vi "PCert-Container-LaunchGlobalDBActor.vi"(8 "error in (no error)":errorcluster, 11 "ERP-Container-UI in":refnum<class "PCert-Container-UI.lvclass">) -> (0 "error out":errorcluster, 3 "ERP-Container-UI out":refnum<class "PCert-Container-UI.lvclass">)   [LabVIEW 2013, in "PCert-Container-UI.lvclass"]
uses:
  PCert-Container-UI.lvclass
  ftw-dataflow/Actor/src/Connector/FTW-ActorConnector.lvclass
  PCert-Container-UI.lvclass/PCert-Container-UI.ctl
  Actors/Database-Actor/PartCertDatabase-Actor.lvclass
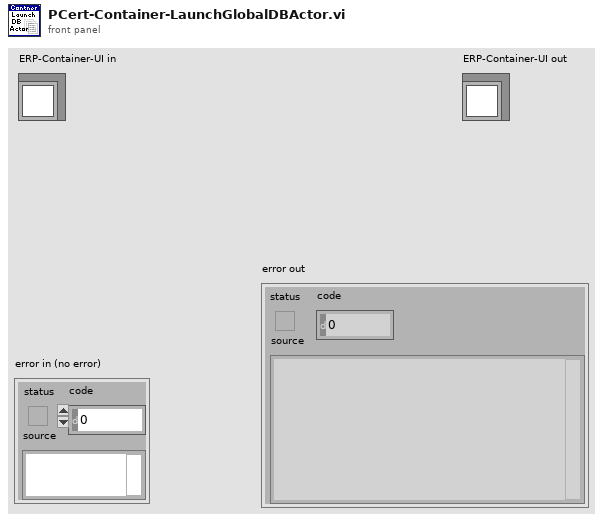
[diagram p1: front panel]
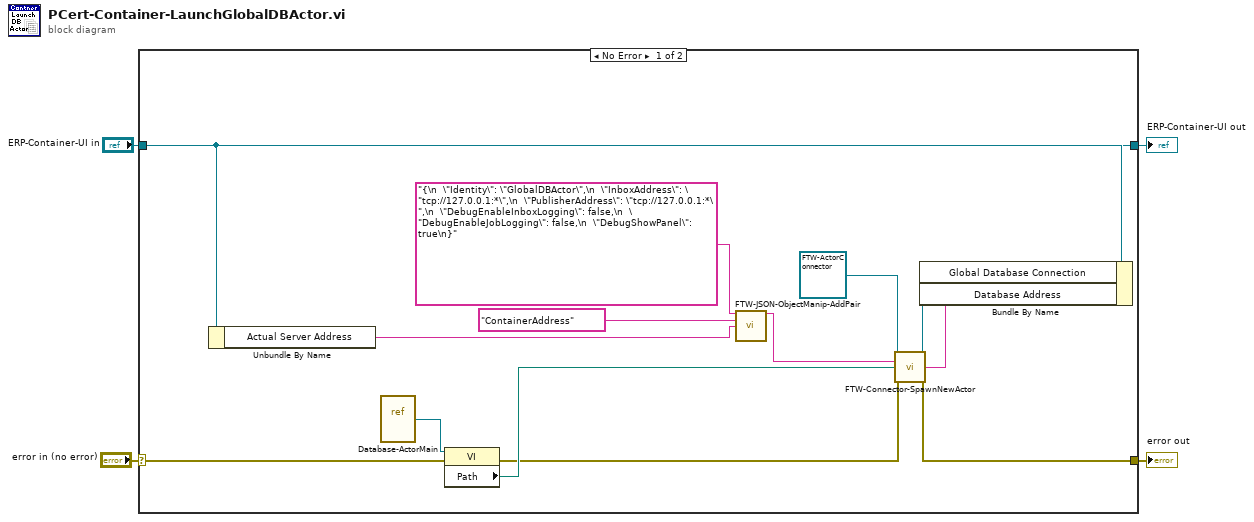
[diagram p0: block diagram]
diagram:
  n1 = case shown="No Error" "error in (no error)" {
    selector: "error in (no error)" -> [w8 w20]
    tunnel: [w10 w20] -> w3
    tunnel: [w12 w19] -> w1
    tunnel: "ERP-Container-UI in" -> [w14 w19]
    frame No Error {
      n2 = Unbundle By Name(w14) -> ("Actual Server Address"=w15:string)
      n3 = vi-ref "Database-ActorMain.vi"() -> (w7:refnum<vi>)
      n4 = property class="VI"(reference=w7, error in=w8) -> (error out=w5:errorcluster, "Path"=w6:path)  [unwired: 1 out]
      n5 = call "FTW-JSON-ObjectManip-AddPair.vi"("Input JSON Object"="{\n  \"Identity\": \"GlobalDBActor\",\n  \"InboxAddress\": \"tcp://127.0.0.1:*\",\n  \"PublisherAddress\": \"tcp://127.0.0.1:*\",\n  \"DebugEnableInboxLogging\": false,\n  \"DebugEnableJobLogging\": false,\n  \"DebugShowPanel\": true\n}" ("Configuration"), "Key"="ContainerAddress", "Value"=w15) -> ("Output JSON Object"=w18:string)  [unwired: 11 in, 1 out]
      n6 = call "FTW-Connector-SpawnNewActor.vi"("FTW Actor Connector Type"=refnum<class "FTW-ActorConnector.lvclass"> refnum ("Featherweight Actor:FTW Actor Connector"), "Configuration"=w18, "Actor VI Filepath"=w6, "error in"=w5) -> ("FTW Actor Connector"=w13:refnum<class "FTW-ActorConnector.lvclass">, "Instance Inbox Address"=w11:string, "error out"=w10:errorcluster)  [unwired: 7 in, 2 out]
      n7 = Bundle By Name(cluster=w14, "Global Database Connection"=w13, "Database Address"=w11) -> (w12:refnum<class "PCert-Container-UI.lvclass">)
    }
    frame Error {
    }
  }
  "error out" <- w3
  "ERP-Container-UI out" <- w1
